vi "Process Data1D.vi"(8 "error in (no error)":errorcluster, 10 "Data1D in":refnum<class "Data1D.lvclass">, 11 "ThresholdProcess1D in":refnum<class "ThresholdProcessor1D.lvclass">) -> (0 "error out":errorcluster, 2 "Data1D out":refnum<class "Data1D.lvclass">, 3 "ThresholdProcess1D out":refnum<class "ThresholdProcessor1D.lvclass">)   [LabVIEW 2014, in "ThresholdProcessor1D.lvclass"]
uses:
  ThresholdProcessor1D.lvclass
  Framework/Model/Data/Data1D/Data1D.lvclass
  ThresholdProcessor1D.lvclass/ThresholdProcessor1D.ctl
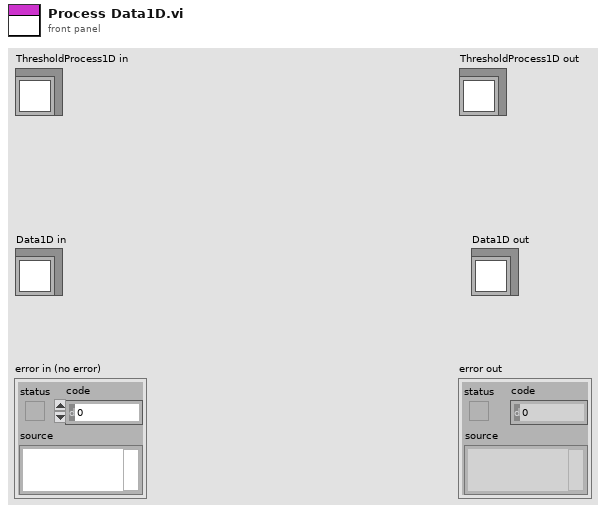
[diagram p1: front panel]
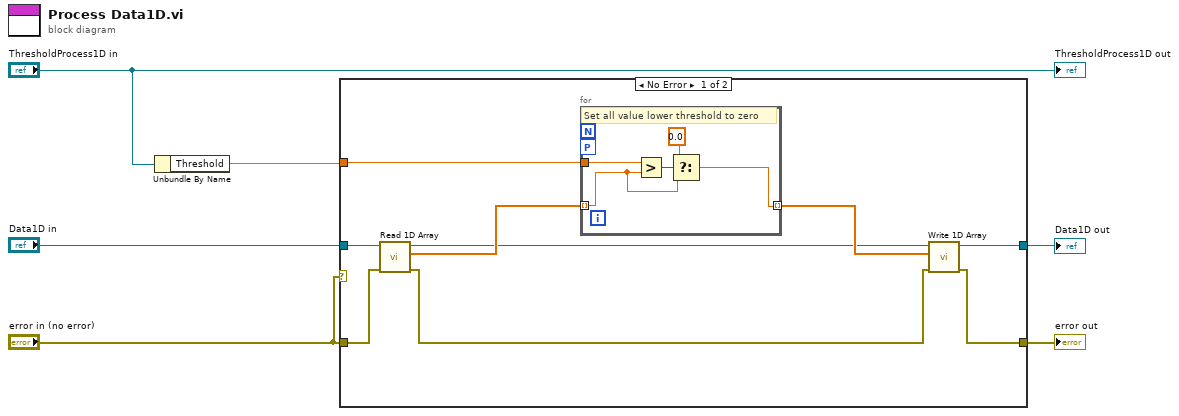
[diagram p0: block diagram]
diagram:
  n1 = Unbundle By Name("ThresholdProcess1D in") -> ("Threshold"=w1:dbl)
  n2 = case shown="No Error" "error in (no error)" {
    tunnel: "error in (no error)" -> [w15 w22]
    tunnel: [w13 w22] -> w6
    tunnel: [w12 w21] -> w3
    tunnel: "Data1D in" -> [w11 w21]
    tunnel: w1 -> [w8 _]
    frame No Error {
      n3 = call "Read 1D Array.vi"("error in (no error)"=w15, "Data1D in"=w11) -> ("error out"=w14:errorcluster, "1D Array"=w10:dbl[], "Data1D out"=w7:refnum<class "Data1D.lvclass">)  [unwired: 7 in]
      n4 = for {
        tunnel: w10 -> [w17] mode=indexing
        tunnel: [w18] -> w9 mode=indexing
        tunnel: w8 -> [w19]
        workers-P: _ -> [_]
        # "Set all value lower threshold to zero"
        n5 = Greater?(x=w19, y=w17) -> (0:w20:bool)
        n6 = Select(t=0.0, s=w20, f=w17) -> (s? t:f=w18:dbl)
      }
      n7 = call "Write 1D Array.vi"("error in (no error)"=w14, "1D Array"=w9, "Data1D in"=w7) -> ("error out"=w13:errorcluster, "Data1D out"=w12:refnum<class "Data1D.lvclass">)  [unwired: 7 in]
    }
    frame Error {
    }
  }
  "error out" <- w6
  "Data1D out" <- w3
  "ThresholdProcess1D out" <- "ThresholdProcess1D in"
